vi "Insert Start Message.vi"(8 "error in (no error)":errorcluster, 10 "Start Time":timestamp, 11 "TrialBasedExperiment in":refnum<class "TrialBasedExperiment.lvclass">) -> (0 "error out":errorcluster, 3 "TrialBasedExperiment out":refnum<class "TrialBasedExperiment.lvclass">)   [LabVIEW 2014, in "AcquisitionCoreObjects.lvlib" / "TrialBasedExperiment.lvclass"]
uses:
  TrialBasedExperiment.lvclass
  Acquisition/Database/StimulationPrimary.ctl
  Acquisition/Database/SessionPrimary.ctl
  Acquisition/AcquistionObject/AcquistionObject.lvclass
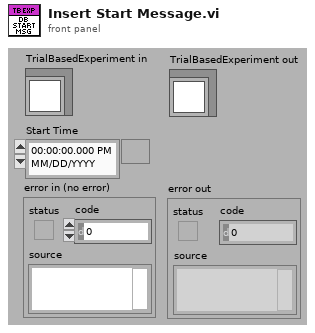
[diagram p1: front panel]
types:
  T1 = typedef "StimulationPrimary.ctl" = cluster{"setup":u8, "subject_id":i32, "session_start_time":dbl, "stim_start_time":dbl}
  T2 = cluster{"setup":u8, "subject_id":i32, "session_start_time":dbl, "stim_start_time":dbl, "stim_path":path, "exp_type":string, "stim_stop_time":dbl}
  T3 = typedef "NI_Database_API.lvlib/Conn ObjectReference.ctl" = refnum<k1>
  T4 = typedef "SessionPrimary.ctl" = cluster{"setup":u8, "subject_id":i32, "session_start_time":dbl}
  T5 = cluster{"reference":T3, "table":string, "columns":string[], i32}
  T6 = cluster{cluster{"reference":T3, "table":string, "columns":string[], i32}, "Variant":variant}
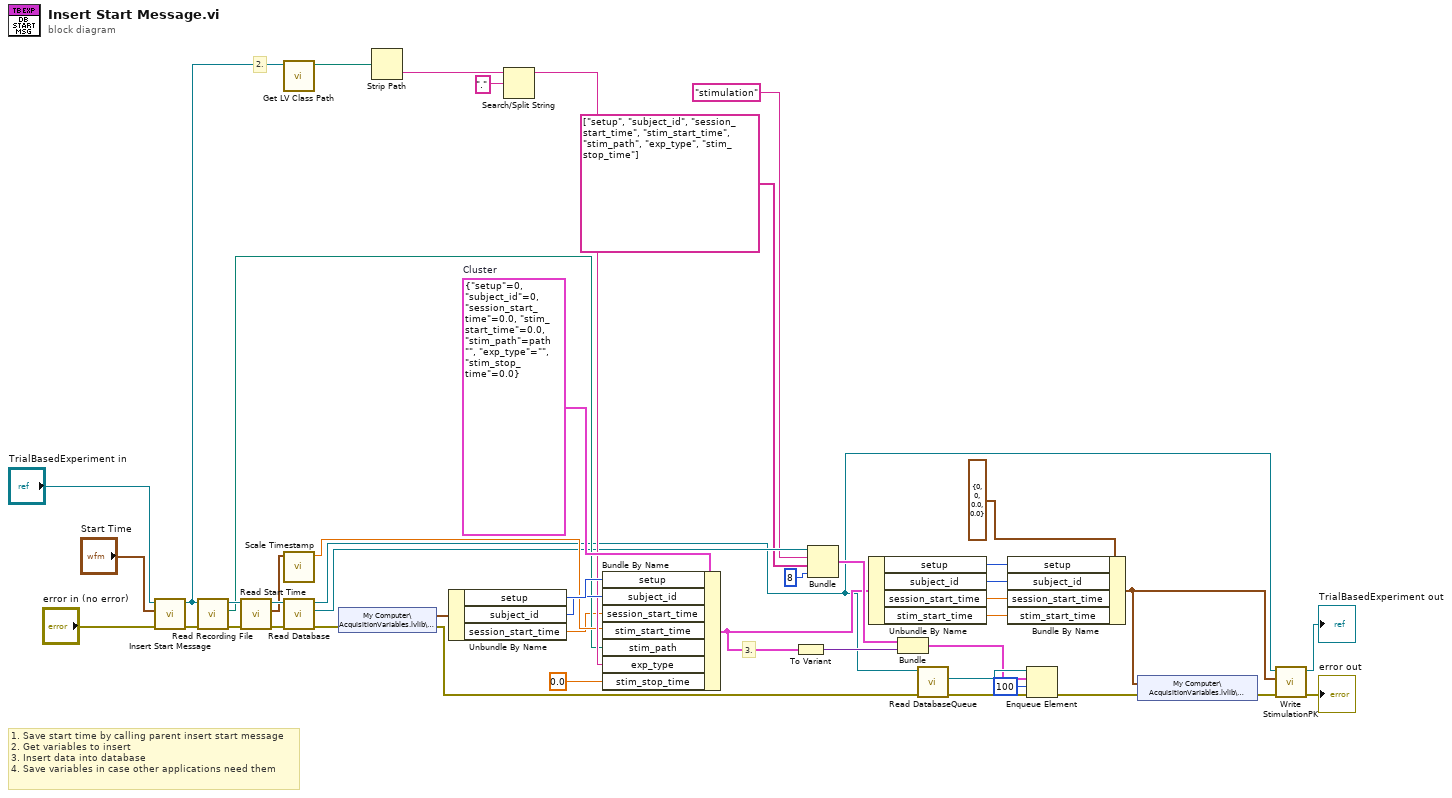
[diagram p0: block diagram]
diagram:
  w43 = T2 {"setup"=0, "subject_id"=0, "session_start_time"=0.0, "stim_start_time"=0.0, "stim_path"=path "", "exp_type"="", "stim_stop_time"=0.0}  # Cluster
  # "2."
  # "3."
  # "1. Save start time by calling parent insert start message\n2. Get variables to insert\n3. Insert data into database\n4. Save variables in case other applications need them"
  n1 = call-parent "Insert Start Message.vi"("error in (no error)"="error in (no error)", "Start Time"="Start Time", "AcquistionObject in"="TrialBasedExperiment in") -> ("error out"=w31:errorcluster, "AcquistionObject out"=w27:refnum<class "TrialBasedExperiment.lvclass">)  [unwired: 7 in]
  n2 = call-dynamic "Read Recording File.vi"("error in (no error)"=w31, "AcquistionObject in"=w27) -> ("error out"=w35:errorcluster, "Recording File"=w23:path, "AcquistionObject out"=w36:refnum<class "TrialBasedExperiment.lvclass">)  [unwired: 7 in]
  n3 = call-dynamic "Read Start Time.vi"("error in (no error)"=w35, "AcquistionObject in"=w36) -> ("error out"=w33:errorcluster, "Start Time"=w25:timestamp, "AcquistionObject out"=w34:refnum<class "TrialBasedExperiment.lvclass">)  [unwired: 7 in]
  n4 = call <vilib>:"Get LV Class Path.vi"("object"=w27) -> ("class path"=w30:path)  [unwired: 9 in, 1 out]
  n5 = call "Scale Timestamp.vi"("Time Stamp"=w25) -> ("Scaled timestamp"=w24:dbl)  [unwired: 10 in]
  n6 = call-dynamic "Read Database.vi"("error in (no error)"=w33, "AcquistionObject in"=w34) -> ("error out"=w32:errorcluster, "reference"=w14:T3, "AcquistionObject out"=w7:refnum<class "TrialBasedExperiment.lvclass">)  [unwired: 7 in]
  n7 = shared-variable "My Computer\\AcquisitionVariables.lvlib\\SessionPK"(error in=w32) -> (w37:T4, error out=w6:errorcluster)
  n8 = Strip Path(path=w30) -> (name=w29:string)  [unwired: 1 out]
  n9 = Unbundle By Name(w37) -> ("setup"=w42:u8, "subject_id"=w41:i32, "session_start_time"=w21:dbl)
  n10 = Search/Split String(string=w29, search string/char (-)=".") -> (substring before match=w26:string)  [unwired: 1 in, 2 out]
  n11 = Bundle By Name(cluster=w43, "setup"=w42, "subject_id"=w41, "session_start_time"=w21, "stim_start_time"=w24, "stim_path"=w23, "exp_type"=w26, "stim_stop_time"=0.0) -> (w9:T2)
  n12 = To Variant(anything=w9) -> (Variant=w8:variant)
  n13 = Bundle("reference"=w14, "table"="stimulation", "columns"=string[] ["setup", "subject_id", "session_start_time", "stim_start_time", "stim_path", "exp_type", "stim_stop_time"], 8) -> (w10:T5)  [unwired: 1 in]
  n14 = Unbundle By Name(w9) -> ("setup"=w40:u8, "subject_id"=w39:i32, "session_start_time"=w38:dbl, "stim_start_time"=w20:dbl)
  n15 = Bundle(w10, "Variant"=w8) -> (w4:T6)  [unwired: 1 in]
  n16 = call-dynamic "Read DatabaseQueue.vi"("error in (no error)"=w6, "AcquistionObject in"=w7) -> ("error out"=w3:errorcluster, "DatabaseQueue"=w5:refnum<queue>)  [unwired: 7 in, 1 out]
  n17 = Bundle By Name(cluster=T1 {"setup"=0, "subject_id"=0, "session_start_time"=0.0, "stim_start_time"=0.0} ("StimulationPK"), "setup"=w40, "subject_id"=w39, "session_start_time"=w38, "stim_start_time"=w20) -> (w19:T1)
  n18 = Enqueue Element(queue=w5, element=w4, timeout in ms (-1)=100, error in (no error)=w3) -> (error out=w2:errorcluster)  [unwired: 2 out]
  n19 = shared-variable "My Computer\\AcquisitionVariables.lvlib\\StimulationPK"(w19, error in=w2) -> (error out=w18:errorcluster)
  n20 = call-dynamic "Write StimulationPK.vi"("error in (no error)"=w18, "StimulationPK"=w19, "TrialBasedExperiment in"=w7) -> ("error out"=→"error out":errorcluster, "TrialBasedExperiment out"=→"TrialBasedExperiment out":refnum<class "TrialBasedExperiment.lvclass">)  [unwired: 7 in]
